vi "Post-Uninstall Custom Action.vi"(10 "Variant":variant) -> (0 "error out":errorcluster)   [LabVIEW 2020]
uses:
  <vilib>/zip/NI_Unzip.lvlib
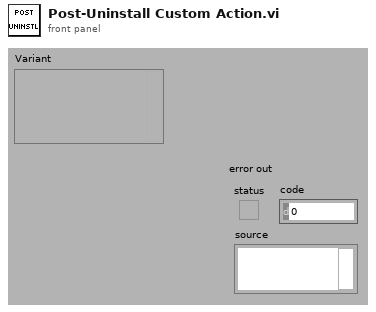
[diagram p1: front panel]
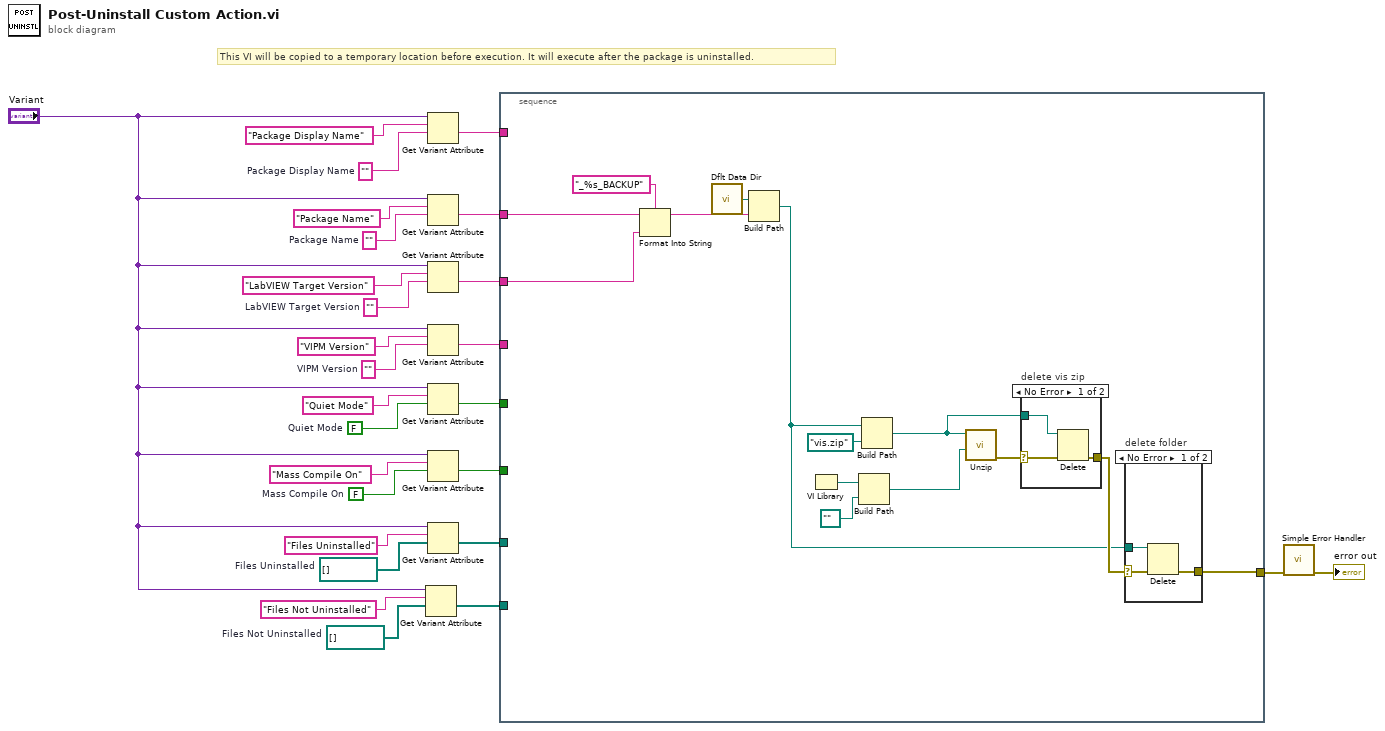
[diagram p0: block diagram]
diagram:
  w3 = path[] []  # Files Not Uninstalled
  w4 = path[] []  # Files Uninstalled
  w10 = FALSE  # Mass Compile On
  w11 = ""  # Package Display Name
  w18 = FALSE  # Quiet Mode
  w21 = ""  # VIPM Version
  w23 = ""  # LabVIEW Target Version
  w25 = ""  # Package Name
  # "This VI will be copied to a temporary location before execution. It will execute after the package is uninstalled."
  n1 = Get Variant Attribute(Variant="Variant", name="Files Not Uninstalled", default value (empty Variant)=w3) -> (value=w8:path[])  [unwired: 1 in, 3 out]
  n2 = Get Variant Attribute(Variant="Variant", name="Package Display Name", default value (empty Variant)=w11) -> (value=w17:string)  [unwired: 1 in, 3 out]
  n3 = Get Variant Attribute(Variant="Variant", name="Package Name", default value (empty Variant)=w25) -> (value=w16:string)  [unwired: 1 in, 3 out]
  n4 = Get Variant Attribute(Variant="Variant", name="LabVIEW Target Version", default value (empty Variant)=w23) -> (value=w15:string)  [unwired: 1 in, 3 out]
  n5 = Get Variant Attribute(Variant="Variant", name="VIPM Version", default value (empty Variant)=w21) -> (value=w14:string)  [unwired: 1 in, 3 out]
  n6 = Get Variant Attribute(Variant="Variant", name="Quiet Mode", default value (empty Variant)=w18) -> (value=w13:bool)  [unwired: 1 in, 3 out]
  n7 = Get Variant Attribute(Variant="Variant", name="Mass Compile On", default value (empty Variant)=w10) -> (value=w12:bool)  [unwired: 1 in, 3 out]
  n8 = Get Variant Attribute(Variant="Variant", name="Files Uninstalled", default value (empty Variant)=w4) -> (value=w7:path[])  [unwired: 1 in, 3 out]
  n9 = stacked-sequence {
    tunnel: w17 -> [_]
    tunnel: w16 -> [w30]
    tunnel: w15 -> [w29]
    tunnel: w14 -> [_]
    tunnel: w13 -> [_]
    tunnel: w12 -> [_]
    tunnel: w7 -> [_]
    tunnel: w8 -> [_]
    tunnel: [w33] -> w2
    frame #0 {
      n10 = Format Into String(format string="_%s_BACKUP", initial string=w30, w29) -> (resulting string=w28:string)  [unwired: 1 in, 1 out]
      n11 = call <vilib>:"Dflt Data Dir.vi"() -> ("App:Default Data Directory"=w41:path)
      n12 = Build Path(base path=w41, name or relative path=w28) -> (appended path=w32:path)
      n13 = VI Library() -> (path=w38:path)
      n14 = Build Path(base path=w38, name or relative path=path "..") -> (appended path=w39:path)
      n15 = Build Path(base path=w32, name or relative path=path "vis.zip") -> (appended path=w34:path)
      n16 = call <vilib>:"Unzip.vi"("Target directory (same as Zip file if empty)"=w39, "Zip file"=w34) -> ("error out"=w37:errorcluster)  [unwired: 7 in, 2 out]
      n17 = case "delete vis zip" shown="No Error" w37 {
        selector: w37 -> [w48 w49]
        tunnel: w34 -> [w47 _]
        tunnel: [w46 w49] -> w36
        frame No Error {
          n18 = Delete(path (use dialog)=w47, error in=w48) -> (error out=w46:errorcluster)  [unwired: 3 in, 2 out]
        }
        frame Error {
        }
      }
      n19 = case "delete folder" shown="No Error" w36 {
        selector: w36 -> [w44 w45]
        tunnel: w32 -> [w43 _]
        tunnel: [w42 w45] -> w33
        frame No Error {
          n20 = Delete(path (use dialog)=w43, error in=w44) -> (error out=w42:errorcluster)  [unwired: 3 in, 2 out]
        }
        frame Error {
        }
      }
    }
  }
  n21 = call <vilib>:"Simple Error Handler.vi"("error in (no error)"=w2) -> ("error out"=→"error out":errorcluster)  [unwired: 4 in, 4 out]
